vi "Test Basic Write_Read.vi"(8 "error in (no error)":errorcluster, 11 "Scalar Channels Testing in":refnum<class "Scalar Channels Testing.lvclass">) -> (0 "error out":errorcluster, 3 "Scalar Channels Testing out":refnum<class "Scalar Channels Testing.lvclass">)   [LabVIEW 2019, in "Scalar Channels Testing.lvclass"]
uses:
  Scalar Channels Testing.lvclass
  C:/Program Files (x86)/National Instruments/LabVIEW 2019/vi.lib/NI/NI VeriStand Development Tools/NI Veristand Test Utilities/VeriStandTestCase/VeriStandTestCase.lvclass
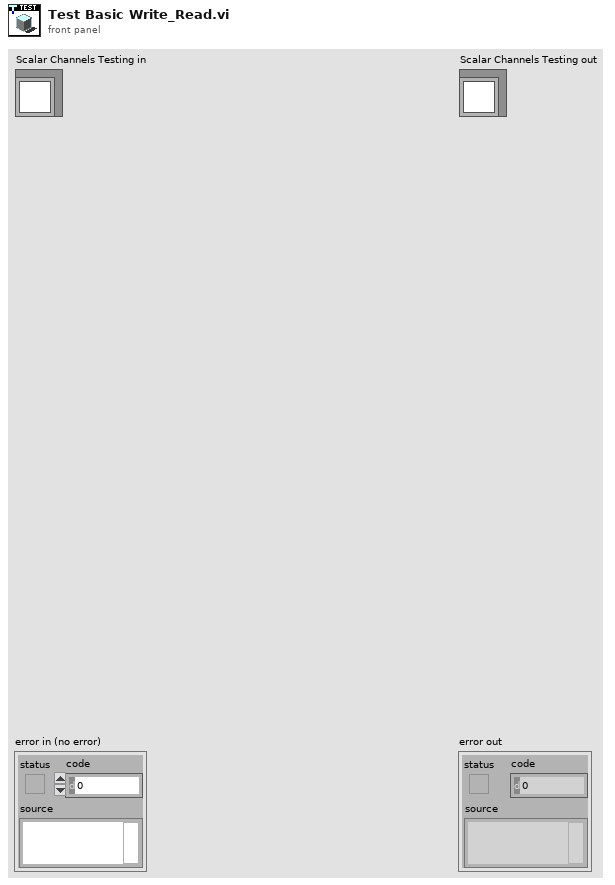
[diagram p1: front panel]
types:
  T1 = typedef "NI_VS Workspace ExecutionAPI.lvlib/WorkspaceAPI.ctl" = refnum<k24>
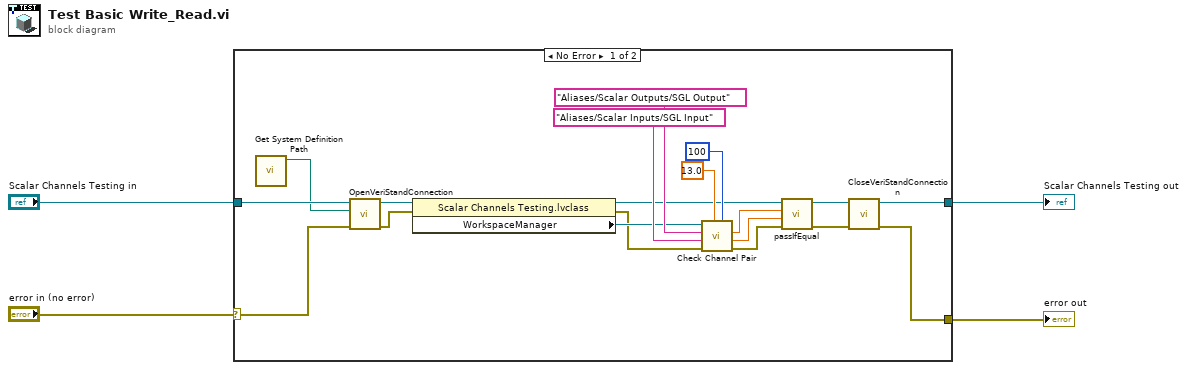
[diagram p0: block diagram]
diagram:
  n1 = case shown="No Error" "error in (no error)" {
    selector: "error in (no error)" -> [w21 w25]
    tunnel: [w20 w25] -> w3
    tunnel: [w22 w24] -> w1
    tunnel: "Scalar Channels Testing in" -> [w23 w24]
    frame No Error {
      n2 = call "Get System Definition Path.vi"() -> ("System Definition path"=w19:path)  [unwired: 11 in]
      n3 = call-dynamic "OpenVeriStandConnection.vi"("error in (no error)"=w21, "System Definition File"=w19, "VeriStand Test Case in"=w23) -> ("error out"=w14:errorcluster, "VeriStand Test Case out"=w13:refnum<class "Scalar Channels Testing.lvclass">)  [unwired: 6 in, 1 out]
      n4 = property class="Scalar Channels Testing.lvclass"(reference=w13, error in=w14) -> (reference out=w10:refnum<class "Scalar Channels Testing.lvclass">, error out=w11:errorcluster, "WorkspaceManager"=w12:T1)
      n5 = call "Check Channel Pair.vi"("milliseconds to wait"=u32 100, "Test Value"=13.0 ("Value"), "error in (no error)"=w11, "Input Channel"="Aliases/Scalar Inputs/SGL Input" ("Channel"), "Output Channel"="Aliases/Scalar Outputs/SGL Output" ("Channel"), "WorkspaceManager in"=w12) -> ("error out"=w6:errorcluster, "InputChannel Value"=w8:dbl, "OutputChannel Value"=w9:dbl)  [unwired: 2 in, 1 out]
      n6 = call-dynamic "passIfEqual.vi"("error in (no error)"=w6, "y"=w8, "x"=w9, "TestCase in"=w10) -> ("error out"=w5:errorcluster, "TestCase out"=w7:refnum<class "Scalar Channels Testing.lvclass">)  [unwired: 6 in]
      n7 = call-dynamic "CloseVeriStandConnection.vi"("error in (no error)"=w5, "VeriStand Test Case in"=w7) -> ("error out"=w20:errorcluster, "VeriStand Test Case out"=w22:refnum<class "Scalar Channels Testing.lvclass">)  [unwired: 8 in]
    }
    frame Error {
    }
  }
  "error out" <- w3
  "Scalar Channels Testing out" <- w1
